vi "Cast Instrument to Instrument Type.vi"(8 "error in (no error)":errorcluster, 9 "Type":T1, 10 "Instrument in":refnum<class "Instrument.lvclass">, 11 "Instrument Classes":T2) -> (0 "error out":errorcluster, 2 "Instrument out":refnum<class "Instrument.lvclass">, 3 "Instrument Classes out":T2)   [LabVIEW 2019, in "Control Experiment.lvclass"]
uses:
  Control Experiment.lvclass
  Typedefs/Instrument Classes--cluster.ctl
  <userlib>/LevyLab/Instrument Framework/Instrument Types/Lockin/Instrument.LockinAPI.lvclass
  <userlib>/LevyLab/Instrument Framework/Instrument Types/Amplifier/Instrument.Amplifier.lvclass
  <userlib>/LevyLab/Instrument Framework/Instrument Types/Cryostat/Instrument.Cryostat.lvclass
  <userlib>/LevyLab/Instrument Framework/Instrument Types/CBridge/Instrument.CBridge.lvclass
  <userlib>/LevyLab/Instrument Framework/Instrument Types/Delay Line/Instrument.DelayLine.lvclass
  <userlib>/LevyLab/Instrument Framework/Instrument Types/Strain/Instrument.Strain.lvclass
  <userlib>/LevyLab/Instrument Framework/Instrument Types/VNA/Instrument.VNA.lvclass
  <userlib>/LevyLab/Instrument Framework/Instrument Types/VSource/Instrument.VSource.lvclass
  Typedefs/Instrument Types--enum.ctl
  <userlib>/LevyLab/Instrument Framework/Instrument/Instrument.lvclass
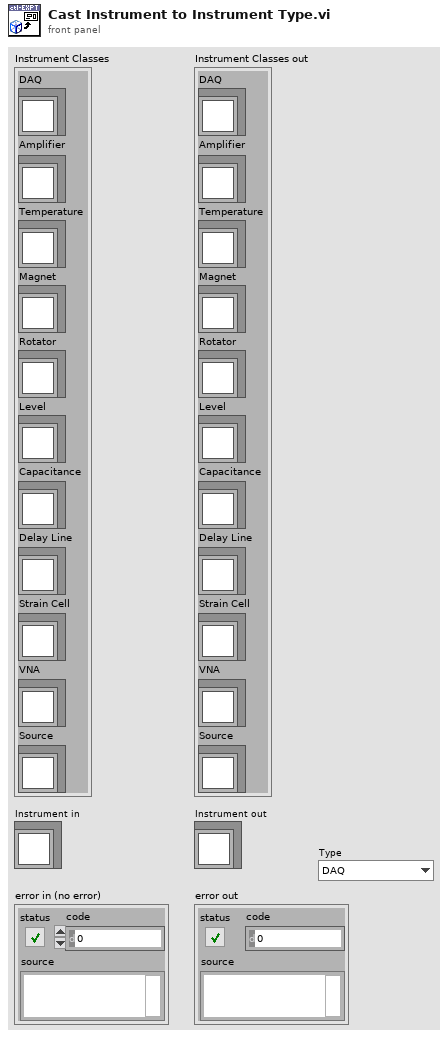
[diagram p1: front panel]
types:
  T1 = typedef "Control Experiment.lvclass/Instrument Types--enum.ctl" = enum16{"DAQ", "Amplifier", "Temperature", "Magnet", "Rotator", "Level", "Capacitance", "Delay Line", "Strain Cell", "VNA", "Source"}
  T2 = typedef "Control Experiment.lvclass/Instrument Classes--cluster.ctl" = cluster{"DAQ":refnum<class "Instrument.LockinAPI.lvclass">, "Amplifier":refnum<class "Instrument.Amplifier.lvclass">, "Temperature":refnum<class "Instrument.Cryostat.lvclass">, "Magnet":refnum<class "Instrument.Cryostat.lvclass">, "Rotator":refnum<class "Instrument.Cryostat.lvclass">, "Level":refnum<class "Instrument.Cryostat.lvclass">, "Capacitance":refnum<class "Instrument.CBridge.lvclass">, "Delay Line":refnum<class "Instrument.DelayLine.lvclass">, "Strain Cell":refnum<class "Instrument.Strain.lvclass">, "VNA":refnum<class "Instrument.VNA.lvclass">, "Source":refnum<class "Instrument.VSource.lvclass">}
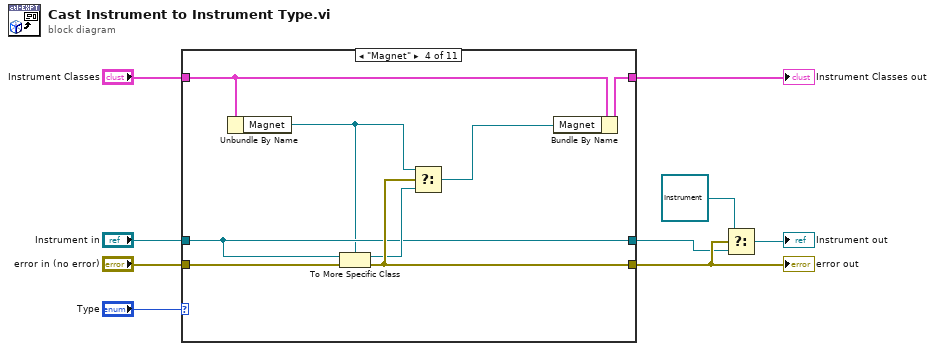
[diagram p0: block diagram]
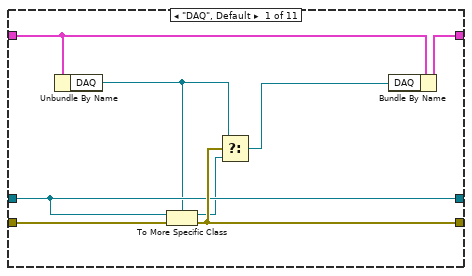
[diagram p2: hidden frame]
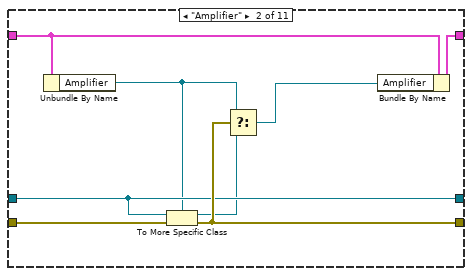
[diagram p3: hidden frame]
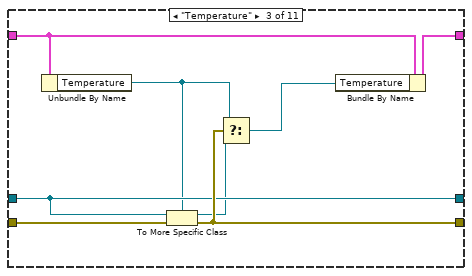
[diagram p4: hidden frame]
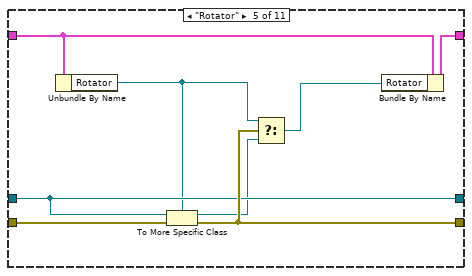
[diagram p5: hidden frame]
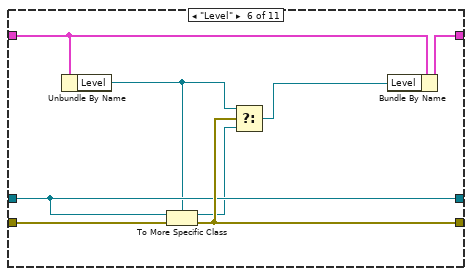
[diagram p6: hidden frame]
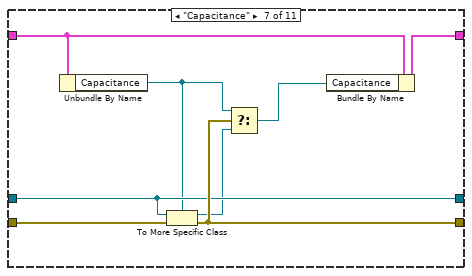
[diagram p7: hidden frame]
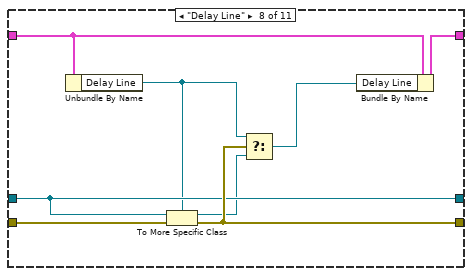
[diagram p8: hidden frame]
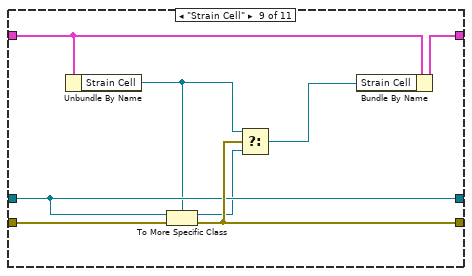
[diagram p9: hidden frame]
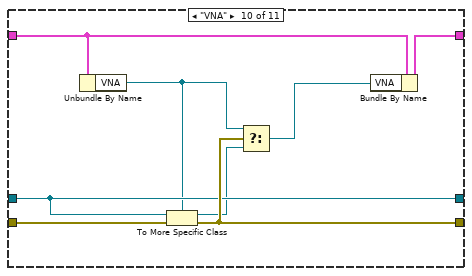
[diagram p10: hidden frame]
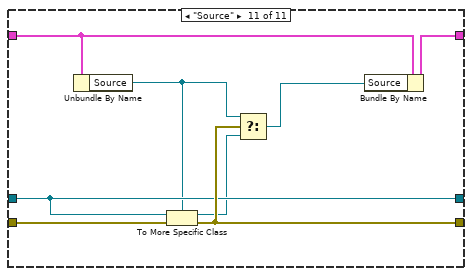
[diagram p11: hidden frame]
diagram:
  n1 = case shown="\"Magnet\"" "Type" {
    tunnel: "Instrument in" -> [w13 w21 w29 w35 w45 w53 w61 w69 w77 w85 w93]
    tunnel: "error in (no error)" -> [w17 w25 w33 w41 w49 w57 w65 w73 w81 w89 w97]
    tunnel: [w14 w22 w30 w38 w46 w54 w62 w70 w78 w86 w94] -> w6
    tunnel: [w13 w21 w29 w35 w45 w53 w61 w69 w77 w85 w93] -> w4
    tunnel: [w15 w23 w31 w39 w47 w55 w63 w71 w79 w87 w95] -> w9
    tunnel: "Instrument Classes" -> [w16 w24 w32 w40 w48 w56 w64 w72 w80 w88 w96]
    frame "DAQ", Default {
      n2 = Unbundle By Name(w16) -> ("DAQ"=w10:refnum<class "Instrument.LockinAPI.lvclass">)
      n3 = To More Specific Class(target class=w10, reference=w13, error in=w17) -> (specific class reference=w12:refnum<class "Instrument.LockinAPI.lvclass">, error out=w14:errorcluster)
      n4 = Select(t=w10, s=w14, f=w12) -> (s? t:f=w11:refnum<class "Instrument.LockinAPI.lvclass">)
      n5 = Bundle By Name(cluster=w16, "DAQ"=w11) -> (w15:T2)
    }
    frame "Amplifier" {
      n6 = Unbundle By Name(w24) -> ("Amplifier"=w19:refnum<class "Instrument.Amplifier.lvclass">)
      n7 = To More Specific Class(target class=w19, reference=w21, error in=w25) -> (specific class reference=w20:refnum<class "Instrument.Amplifier.lvclass">, error out=w22:errorcluster)
      n8 = Select(t=w19, s=w22, f=w20) -> (s? t:f=w18:refnum<class "Instrument.Amplifier.lvclass">)
      n9 = Bundle By Name(cluster=w24, "Amplifier"=w18) -> (w23:T2)
    }
    frame "Temperature" {
      n10 = Unbundle By Name(w32) -> ("Temperature"=w26:refnum<class "Instrument.Cryostat.lvclass">)
      n11 = To More Specific Class(target class=w26, reference=w29, error in=w33) -> (specific class reference=w28:refnum<class "Instrument.Cryostat.lvclass">, error out=w30:errorcluster)
      n12 = Select(t=w26, s=w30, f=w28) -> (s? t:f=w27:refnum<class "Instrument.Cryostat.lvclass">)
      n13 = Bundle By Name(cluster=w32, "Temperature"=w27) -> (w31:T2)
    }
    frame "Magnet" {
      n14 = Unbundle By Name(w40) -> ("Magnet"=w34:refnum<class "Instrument.Cryostat.lvclass">)
      n15 = To More Specific Class(target class=w34, reference=w35, error in=w41) -> (specific class reference=w37:refnum<class "Instrument.Cryostat.lvclass">, error out=w38:errorcluster)
      n16 = Select(t=w34, s=w38, f=w37) -> (s? t:f=w36:refnum<class "Instrument.Cryostat.lvclass">)
      n17 = Bundle By Name(cluster=w40, "Magnet"=w36) -> (w39:T2)
    }
    frame "Rotator" {
      n18 = Unbundle By Name(w48) -> ("Rotator"=w42:refnum<class "Instrument.Cryostat.lvclass">)
      n19 = To More Specific Class(target class=w42, reference=w45, error in=w49) -> (specific class reference=w44:refnum<class "Instrument.Cryostat.lvclass">, error out=w46:errorcluster)
      n20 = Select(t=w42, s=w46, f=w44) -> (s? t:f=w43:refnum<class "Instrument.Cryostat.lvclass">)
      n21 = Bundle By Name(cluster=w48, "Rotator"=w43) -> (w47:T2)
    }
    frame "Level" {
      n22 = Unbundle By Name(w56) -> ("Level"=w51:refnum<class "Instrument.Cryostat.lvclass">)
      n23 = To More Specific Class(target class=w51, reference=w53, error in=w57) -> (specific class reference=w52:refnum<class "Instrument.Cryostat.lvclass">, error out=w54:errorcluster)
      n24 = Select(t=w51, s=w54, f=w52) -> (s? t:f=w50:refnum<class "Instrument.Cryostat.lvclass">)
      n25 = Bundle By Name(cluster=w56, "Level"=w50) -> (w55:T2)
    }
    frame "Capacitance" {
      n26 = Unbundle By Name(w64) -> ("Capacitance"=w58:refnum<class "Instrument.CBridge.lvclass">)
      n27 = To More Specific Class(target class=w58, reference=w61, error in=w65) -> (specific class reference=w60:refnum<class "Instrument.CBridge.lvclass">, error out=w62:errorcluster)
      n28 = Select(t=w58, s=w62, f=w60) -> (s? t:f=w59:refnum<class "Instrument.CBridge.lvclass">)
      n29 = Bundle By Name(cluster=w64, "Capacitance"=w59) -> (w63:T2)
    }
    frame "Delay Line" {
      n30 = Unbundle By Name(w72) -> ("Delay Line"=w68:refnum<class "Instrument.DelayLine.lvclass">)
      n31 = To More Specific Class(target class=w68, reference=w69, error in=w73) -> (specific class reference=w66:refnum<class "Instrument.DelayLine.lvclass">, error out=w70:errorcluster)
      n32 = Select(t=w68, s=w70, f=w66) -> (s? t:f=w67:refnum<class "Instrument.DelayLine.lvclass">)
      n33 = Bundle By Name(cluster=w72, "Delay Line"=w67) -> (w71:T2)
    }
    frame "Strain Cell" {
      n34 = Unbundle By Name(w80) -> ("Strain Cell"=w75:refnum<class "Instrument.Strain.lvclass">)
      n35 = To More Specific Class(target class=w75, reference=w77, error in=w81) -> (specific class reference=w76:refnum<class "Instrument.Strain.lvclass">, error out=w78:errorcluster)
      n36 = Select(t=w75, s=w78, f=w76) -> (s? t:f=w74:refnum<class "Instrument.Strain.lvclass">)
      n37 = Bundle By Name(cluster=w80, "Strain Cell"=w74) -> (w79:T2)
    }
    frame "VNA" {
      n38 = Unbundle By Name(w88) -> ("VNA"=w83:refnum<class "Instrument.VNA.lvclass">)
      n39 = To More Specific Class(target class=w83, reference=w85, error in=w89) -> (specific class reference=w84:refnum<class "Instrument.VNA.lvclass">, error out=w86:errorcluster)
      n40 = Select(t=w83, s=w86, f=w84) -> (s? t:f=w82:refnum<class "Instrument.VNA.lvclass">)
      n41 = Bundle By Name(cluster=w88, "VNA"=w82) -> (w87:T2)
    }
    frame "Source" {
      n42 = Unbundle By Name(w96) -> ("Source"=w91:refnum<class "Instrument.VSource.lvclass">)
      n43 = To More Specific Class(target class=w91, reference=w93, error in=w97) -> (specific class reference=w90:refnum<class "Instrument.VSource.lvclass">, error out=w94:errorcluster)
      n44 = Select(t=w91, s=w94, f=w90) -> (s? t:f=w92:refnum<class "Instrument.VSource.lvclass">)
      n45 = Bundle By Name(cluster=w96, "Source"=w92) -> (w95:T2)
    }
  }
  "error out" <- w6
  "Instrument Classes out" <- w9
  n46 = Select(t=refnum<class "Instrument.lvclass"> refnum ("Instrument out"), s=w6, f=w4) -> (s? t:f=→"Instrument out":refnum<class "Instrument.lvclass">)
